vi "BuildFarm Directory.vi"() -> (0 "BuildFarm Directory":path)   [LabVIEW 2017]
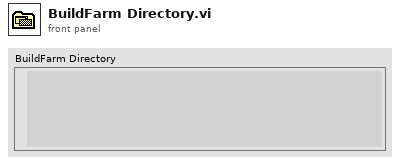
[diagram p1: front panel]
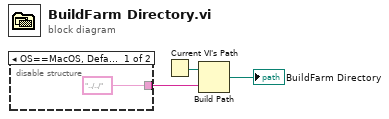
[diagram p0: block diagram]
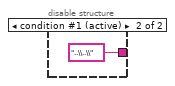
[diagram p2: hidden frame]
diagram:
  n1 = disable-structure shown="OS==MacOS, Default" {
    disable-tunnel: ["../../" ("name or relative path") "..\\..\\" ("name or relative path")] -> w1
    frame condition #0 {
    }
    frame condition #1 (active) {
    }
  }
  n2 = Current VI's Path() -> (path=w3:path)
  n3 = Build Path(base path=w3, name or relative path=w1) -> (appended path=→"BuildFarm Directory":path)
